vi "4motorDriveCheesyStrafe.vi"(0 "Throttle":dbl(slide) scale=-1.0..1.0, 1 "Steering":dbl(slide) scale=-1.0..1.0, 3 "Strafing":dbl(slide) scale=-1.0..1.0, 5 "Gear":bool) -> (14 "leftMotors":dbl(slide) scale=-1.0..1.0, 16 "rightMotors":dbl(slide) scale=-1.0..1.0)   [LabVIEW 2013]
panel:
  in  "highFast":dbl=0.8
  out "WheelOutsideOfRange":bool
  out "ThrottleOutsideOfRange":bool
  out "Difference":dbl
  in  "# of Filter Steps (teleop at 40 ms)":dbl=5.0
  in  "lowFast":dbl=0.8
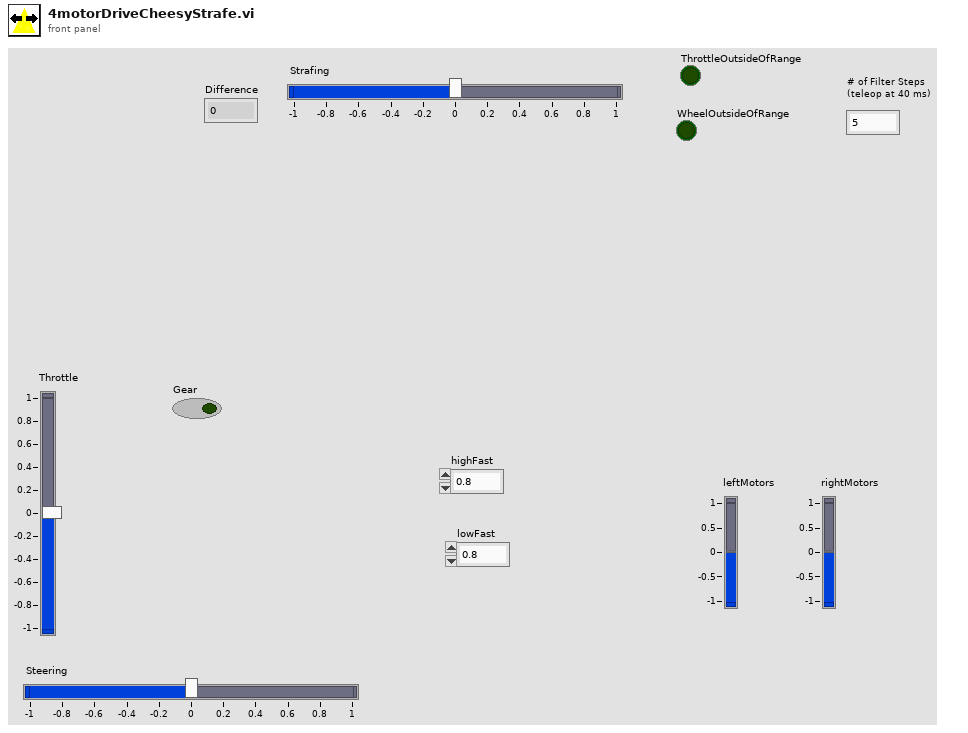
[diagram p1: front panel]
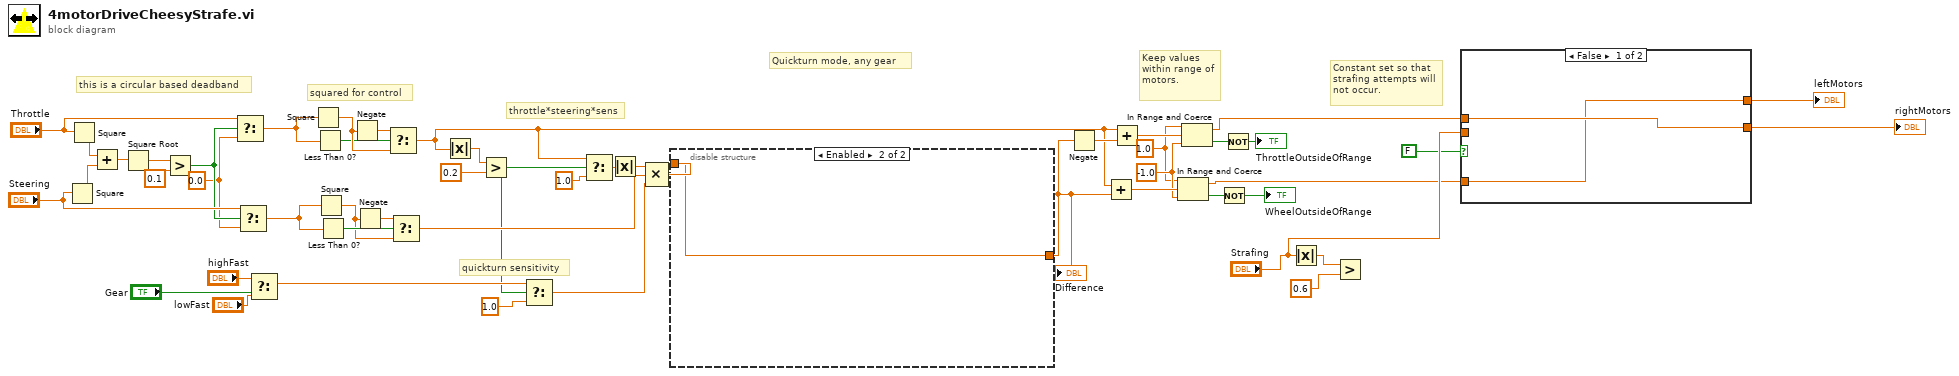
[diagram p0: block diagram]
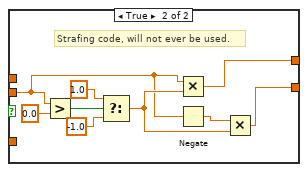
[diagram p2: hidden frame]
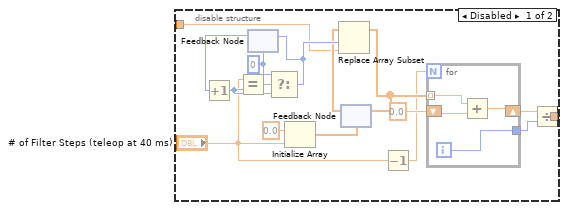
[diagram p3: hidden frame]
diagram:
  w16 = -1.0 ("upper limit")
  w1 = 1.0 ("upper limit")
  w33 = 0.0 ("f")
  # "Keep values within range of motors."
  # "Constant set so that strafing attempts will not occur."
  # "throttle*steering*sens"
  # "squared for control"
  # "quickturn sensitivity"
  # "this is a circular based deadband"
  # "Quickturn mode, any gear"
  n1 = Square(x="Steering") -> (x^2=w38:dbl)
  n2 = Square(x="Throttle") -> (x^2=w39:dbl)
  n3 = Add(x=w39, y=w38) -> (x+y=w37:dbl)
  n4 = Square Root(x=w37) -> (sqrt(x)=w36:dbl)
  n5 = Greater?(x=w36, y=0.1) -> (0:w34:bool)
  n6 = Select(t="Throttle", s=w34, f=w33) -> (s? t:f=w25:dbl)
  n7 = Select(t="Steering", s=w34, f=w33) -> (s? t:f=w32:dbl)
  n8 = Select(t="highFast", s="Gear", f="lowFast") -> (s? t:f=w40:dbl)
  n9 = Square(x=w25) -> (x^2=w27:dbl)
  n10 = Less Than 0?(x=w25) -> (x < 0?=w26:bool)
  n11 = Square(x=w32) -> (x^2=w30:dbl)
  n12 = Less Than 0?(x=w32) -> (x < 0?=w31:bool)
  n13 = Negate(x=w27) -> (-x=w28:dbl)
  n14 = Negate(x=w30) -> (-x=w29:dbl)
  n15 = Select(t=w28, s=w26, f=w27) -> (s? t:f=w11:dbl)
  n16 = Select(t=w29, s=w31, f=w30) -> (s? t:f=w24:dbl)
  n17 = Absolute Value(x=w11) -> (abs(x)=w46:dbl)
  n18 = Greater?(x=w46, y=0.2) -> (0:w15:bool)
  n19 = Select(t=w40, s=w15, f=1.0) -> (s? t:f=w23:dbl)
  n20 = Select(t=w11, s=w15, f=1.0) -> (s? t:f=w13:dbl)
  n21 = Absolute Value(x=w13) -> (abs(x)=w4:dbl)
  n22 = Compound Arithmetic op=MULTIPLY(w4, w24, w23) -> (w12:dbl)
  n23 = disable-structure shown="Enabled" {
    disable-tunnel: [w53 w71] -> w45
    disable-tunnel: w12 -> [w51 w71]
    frame Disabled {
      w63 = 0
      n24 = feedback #1(w63) -> (w59:i32)
      n25 = Increment(x=w59) -> (x+1=w57:i32)
      n26 = Equal?(x="# of Filter Steps (teleop at 40 ms)", y=w57) -> (x = y?=w56:bool)
      n27 = Select(t=w63, s=w56, f=w57) -> (s? t:f=w64:i32)
      n28 = feedback-in #1(w64) -> ()
      n29 = Initialize Array(0.0 ("element"), "# of Filter Steps (teleop at 40 ms)") -> (w55:dbl[])
      n30 = feedback #2(w55) -> (w58:dbl[])
      n31 = Replace Array Subset(array=w58, new element=w51, index=w64) -> (w62:dbl[])
      n32 = feedback-in #2(w62) -> ()
      n33 = Decrement(x="# of Filter Steps (teleop at 40 ms)") -> (x-1=w60:dbl)
      n34 = for {
        N: w60 -> [_]
        tunnel: w62 -> [w68] mode=indexing
        shift-right: [w70] -> w65
        shift-left: 0.0 ("element") -> [w69]
        tunnel: [w67] -> w66
        i -> [w67]
        n35 = Add(x=w68, y=w69) -> (x+y=w70:dbl)
      }
      n36 = Divide(x=w65, y=w66) -> (x/y=w53:dbl)
    }
    frame Enabled {
    }
  }
  "Difference" <- w45
  n37 = Negate(x=w45) -> (-x=w47:dbl)
  n38 = Add(x=w11, y=w45) -> (x+y=w17:dbl)
  n39 = Add(x=w11, y=w47) -> (x+y=w22:dbl)
  n40 = In Range and Coerce(upper limit=w1, x=w17, lower limit=w16) -> (coerced(x)=w6:dbl, In Range?=w18:bool)
  n41 = In Range and Coerce(upper limit=w1, x=w22, lower limit=w16) -> (coerced(x)=w7:dbl, In Range?=w21:bool)
  n42 = Not(x=w18) -> (.not. x?=→"WheelOutsideOfRange":bool)
  n43 = Not(x=w21) -> (.not. x?=→"ThrottleOutsideOfRange":bool)
  n44 = Absolute Value(x="Strafing") -> (abs(x)=w10:dbl)
  n45 = Greater?(x=w10, y=0.6) -> ()  [unwired: 1 out]
  n46 = case shown="False" FALSE {
    tunnel: "Strafing" -> [_ w77]
    tunnel: [w73 w75] -> w2
    tunnel: [w72 w74] -> w3
    tunnel: w7 -> [w73 _]
    tunnel: w6 -> [w72 _]
    frame False {
    }
    frame True {
      # "Strafing code, will not ever be used."
      n47 = Greater?(x=w77, y=0.0) -> (0:w81:bool)
      n48 = Select(t=1.0, s=w81, f=-1.0) -> (s? t:f=w78:dbl)
      n49 = Multiply(x=w77, y=w78) -> (x*y=w74:dbl)
      n50 = Negate(x=w77) -> (-x=w76:dbl)
      n51 = Multiply(x=w76, y=w78) -> (x*y=w75:dbl)
    }
  }
  "leftMotors" <- w3
  "rightMotors" <- w2
